vi "ReplayFrame.vi"(8 "error in (no error)":errorcluster, 11 "DemoCamera in":refnum<class "DemoCamera.lvclass">) -> (0 "error out":errorcluster, 3 "DemoCamera out":refnum<class "DemoCamera.lvclass">)   [LabVIEW 2020, in "DemoCamera.lvlib" / "DemoCamera.lvclass"]
uses:
  DemoCamera.lvclass
  Hardware Abstraction Layer/Component/Device/Device/DeviceStatus.ctl
  Hardware Abstraction Layer/Component/Device/Device/Device.lvlib
panel:
  in  "FrameId":dbl format="%#_13g"
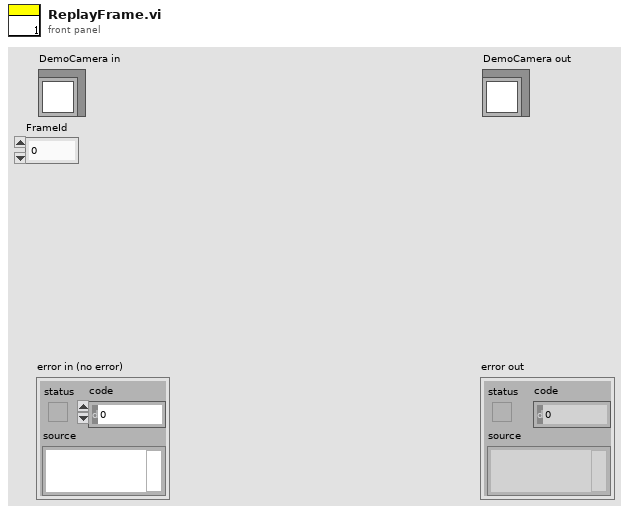
[diagram p1: front panel]
types:
  T1 = typedef "Device.lvlib/DeviceStatus.ctl" = i32
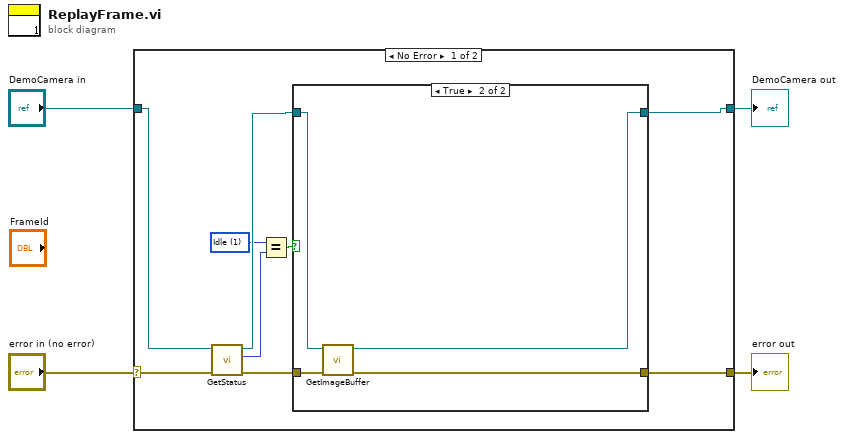
[diagram p0: block diagram]
diagram:
  n1 = case shown="No Error" "error in (no error)" {
    selector: "error in (no error)" -> [w13 w21]
    tunnel: [w11 w21] -> w3
    tunnel: [w9 w20] -> w1
    tunnel: "DemoCamera in" -> [w12 w20]
    frame No Error {
      w7 = T1 1 items=["Offline", "Idle", "Busy"] ("x")
      n2 = call-dynamic "GetStatus.vi"("error in (no error)"=w13, "Device in"=w12) -> ("error out"=w5:errorcluster, "Status"=w8:T1, "Device out"=w10:refnum<class "DemoCamera.lvclass">)  [unwired: 7 in]
      n3 = Equal?(x=w7, y=w8) -> (x = y?=w6:bool)
      n4 = case shown="True" w6 {
        tunnel: [w14 w18] -> w11
        tunnel: w10 -> [w15 w17]
        tunnel: [w15 w16] -> w9
        tunnel: w5 -> [w14 w19]
        frame False {
        }
        frame True {
          n5 = call-dynamic "GetImageBuffer.vi"("error in (no error)"=w19, "Camera in"=w17) -> ("error out"=w18:errorcluster, "Camera out"=w16:refnum<class "DemoCamera.lvclass">)  [unwired: 6 in, 2 out]
        }
      }
    }
    frame Error {
    }
  }
  "error out" <- w3
  "DemoCamera out" <- w1
